vi "Autonomous Independent.vi"() -> ()   [LabVIEW 2019]
doc: "This VI is called when autonomous begins, and will automatically be terminated when autonomous ends. You can carry out timed or sensor driven robot movement independently without needing to return to the caller."
uses:
  <vilib>/Rock Robotics/Network Tables/NT Read String.vi
  Drive/Drive Global.vi
  Shoot/Shoot Global.vi
  Intake/Intake Global.vi
  Index/Index Global.vi
panel:
  in  "Timeout Threshold (ms)":dbl
  # "Be sure to right-click and choose Data Operations>>Make Current Value default if you want to save the array values with the VI"
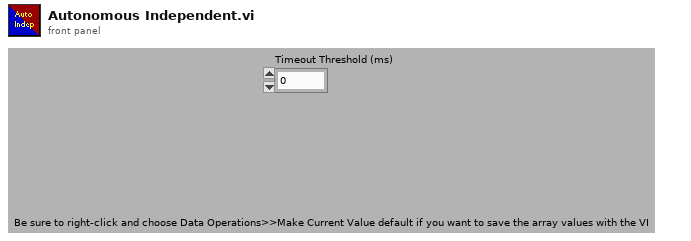
[diagram p1: front panel]
types:
  T1 = typedef "Drive Command Typedef.ctl" = cluster{"Drive Mode":T2, "LeftValue(%)/ relative Distance[u]":dbl, "Right Motor Value(%)/ absolute angle (deg)":dbl, "Timestamp (ms)":dbl}
  T2 = typedef "Drive Mode Typedef.ctl" = enum16{"Disabled", "Auto-align", "Drive Distance", "Turn to angle", "Driver"}
  T3 = typedef "Shooter Command Type Def.ctl" = cluster{"Shooter Mode":T4, "Throttle (%)/ \nSetpoint (RPM)":dbl, "Timestamp (ms)":dbl}
  T4 = typedef "Shooter Mode Type Def.ctl" = enum16{"Disabled", "Raw Throttle", "Velocity Control"}
  T5 = typedef "Intake Command Type Def.ctl" = cluster{"Intake Mode":T6, "Throttle (%)":dbl, "Pneumatic State":T7}
  T6 = typedef "Intake Mode Type Def.ctl" = enum16{"Disabled", "Enabled"}
  T7 = typedef "WPI_SolenoidValue.ctl" = enum16{"Off", "On", "Forward", "Reverse"}
  T8 = cluster{"Drive Command":T1, "Shoot Auton Command":T3, "Intake Command":T5, "Index Motor Values":dbl}[]
  T9 = typedef "Is command done typedef.ctl" = cluster{"Done?":bool, "Timestamp [ms]":dbl}
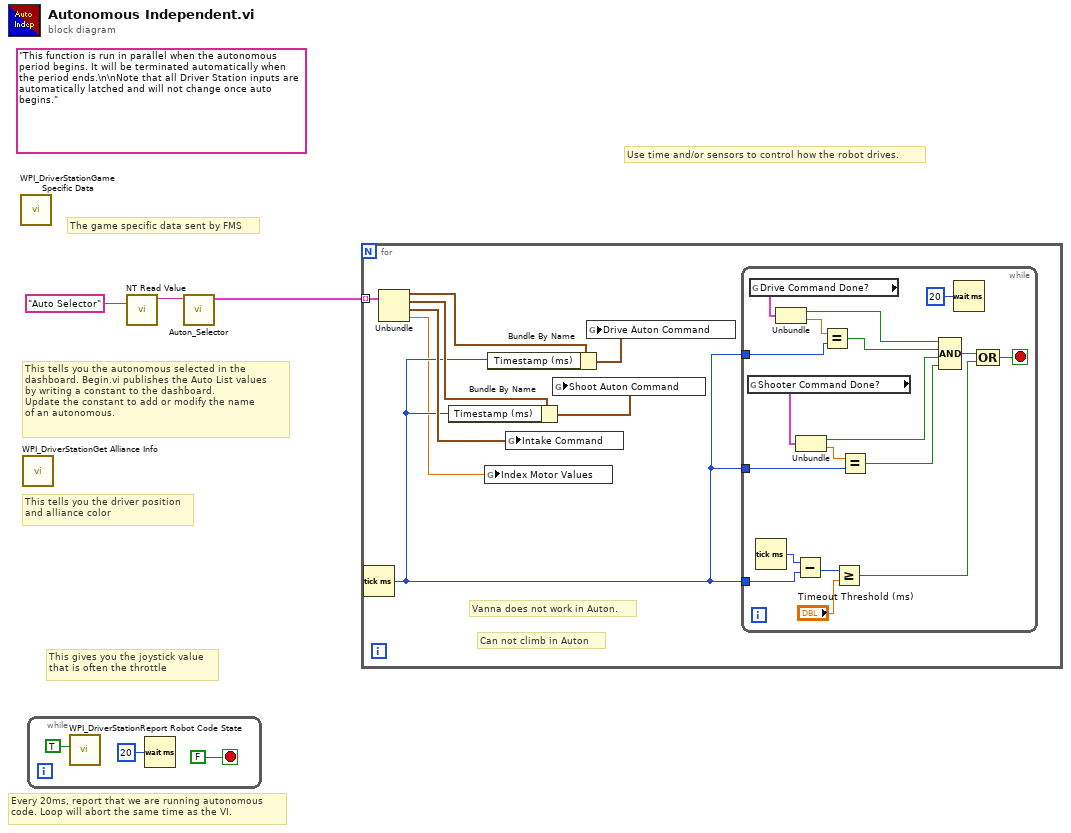
[diagram p0: block diagram]
diagram:
  (unwired) "This function is run in parallel when the autonomous period begins. It will be terminated automatically when the period ends.\n\nNote that all Driver Station inputs are automatically latched and will not change once auto begins."
  # "The game specific data sent by FMS"
  # "This tells you the autonomous selected in the \ndashboard. Begin.vi publishes the Auto List values\nby writing a constant to the dashboard.\nUpdate the constant to add or modify the name\nof an autonomous."
  # "Every 20ms, report that we are running autonomous\ncode. Loop will abort the same time as the VI."
  # "This gives you the joystick value\nthat is often the throttle"
  # "Use time and/or sensors to control how the robot drives."
  # "This tells you the driver position\nand alliance color"
  n1 = call <vilib>:"WPI_DriverStationGame Specific Data.vi"() -> ()  [unwired: 11 in, 1 out]
  n2 = call <vilib>:"WPI_DriverStationGet Alliance Info.vi"() -> ()  [unwired: 12 out]
  n3 = while {
    stop <- FALSE stop-if-true
    n4 = call <vilib>:"WPI_DriverStationReport Robot Code State.vi"("Autonomous"=TRUE) -> ()  [unwired: 10 in, 1 out]
    n5 = Wait (ms)(milliseconds to wait=u32 20) -> ()  [unwired: 1 out]
  }
  n6 = call-poly <vilib>:"NT Read Value.vi"("Name"="Auto Selector") -> ("String"=w2:string)  [unwired: 9 in, 1 out]
  n7 = call "Auton_Selector.vi"("Auton Name In"=w2) -> ("Auton Steps"=w1:T8)  [unwired: 10 in]
  n8 = for {
    tunnel: w1 -> [w14] mode=indexing
    # "Can not climb in Auton"
    # "Vanna does not work in Auton."
    n9 = Tick Count (ms)() -> (millisecond timer value=w8:u32)
    n10 = Unbundle(w14) -> ("Drive Command"=w12:T1, "Shoot Auton Command"=w11:T3, "Intake Command"=w9:T5, "Index Motor Values"=w7:dbl)
    n11 = Bundle By Name(cluster=w11, "Timestamp (ms)"=w8) -> (w10:T3)
    n12 = global write "Index Global.vi" "Index Motor Values"(w7) -> ()
    n13 = Bundle By Name(cluster=w12, "Timestamp (ms)"=w8) -> (w13:T1)
    n14 = global write "Intake Global.vi" "Intake Command"(w9) -> ()
    n15 = global write "Shoot Global.vi" "Shoot Auton Command"(w10) -> ()
    n16 = global write "Drive Global.vi" "Drive Auton Command"(w13) -> ()
    n17 = while {
      tunnel: w8 -> [w25]
      tunnel: w8 -> [w30]
      tunnel: w8 -> [w18]
      stop <- w27 stop-if-true
      n18 = global read "Shoot Global.vi" "Shooter Command Done?"() -> (w15:T9)
      n19 = global read "Drive Global.vi" "Drive Command Done?"() -> (w16:T9)
      n20 = Tick Count (ms)() -> (millisecond timer value=w31:u32)
      n21 = Unbundle(w16) -> ("Done?"=w23:bool, "Timestamp [ms]"=w24:dbl)
      n22 = Subtract(x=w31, y=w30) -> (x-y=w29:u32)
      n23 = Unbundle(w15) -> ("Done?"=w20:bool, "Timestamp [ms]"=w19:dbl)
      n24 = Equal?(x=w24, y=w25) -> (x = y?=w22:bool)
      n25 = Greater Or Equal?(x=w29, y="Timeout Threshold (ms)") -> (x >= y?=w21:bool)
      n26 = Equal?(x=w19, y=w18) -> (x = y?=w17:bool)
      n27 = Compound Arithmetic op=AND(w23, w22, w20, w17) -> (w26:bool)
      n28 = Wait (ms)(milliseconds to wait=u32 20) -> ()  [unwired: 1 out]
      n29 = Compound Arithmetic op=OR(w26, w21) -> (w27:bool)
    }
  }
